vi "Control PID.vi"(5 "action":enum16{"CHECK", "INIT"}(ring), 6 "ITC temperature":dbl, 7 "time (sec)":dbl=3600.0, 8 "error in":errorcluster, 9 "Pid control":T1={" PID table "=[[400.0, 10.0, 3.0, 1.0], [300.0, 10.0, 3.0, 1.0], [60.0, 10.0, 3.0, 1.0], [40.0, 10.0, 3.0, 1.0], [20.0, 30.0, 0.5, 0.2], [10.0, 40.0, 0.5, 0.2], [1.0, 50.0, 0.2, 0.2], [0.0, 50.0, 0.2, 0.2]], "PID update interval (min)"=3600, "(mins) since PID update "=5.0, "P"=10.0, "I"=3.0, "D"=1.0, "PID is"=TRUE} {"D" format="%.2f"; "I" format="%.2f"; "P" format="%.2f"; "(mins) since PID update" format="%_3f"}) -> (0 "error out":errorcluster, 1 "Pid control Out":T1={" PID table "=[[400.0, 10.0, 3.0, 1.0], [300.0, 10.0, 3.0, 1.0], [60.0, 10.0, 3.0, 1.0], [40.0, 10.0, 3.0, 1.0], [20.0, 30.0, 0.5, 0.2], [10.0, 40.0, 0.5, 0.2], [1.0, 50.0, 0.2, 0.2], [0.0, 50.0, 0.2, 0.2]], "PID update interval (min)"=3600, "(mins) since PID update "=5.0, "P"=10.0, "I"=3.0, "D"=1.0, "PID is"=TRUE} {"D" format="%.2f"; "I" format="%.2f"; "P" format="%.2f"; "(mins) since PID update" format="%_3f"})   [LabVIEW 2012]
uses:
  Pid control.ctl
  itc 503 box - control.ctl
  Q -- check range -- i -- real.vi
  Q - not nan and gtr than zero - Real.vi
  Q - not nan -- real.vi
panel:
  # "Temp (K)                  P                          I                         D"
  # "Temp (K)                  P                          I                         D"
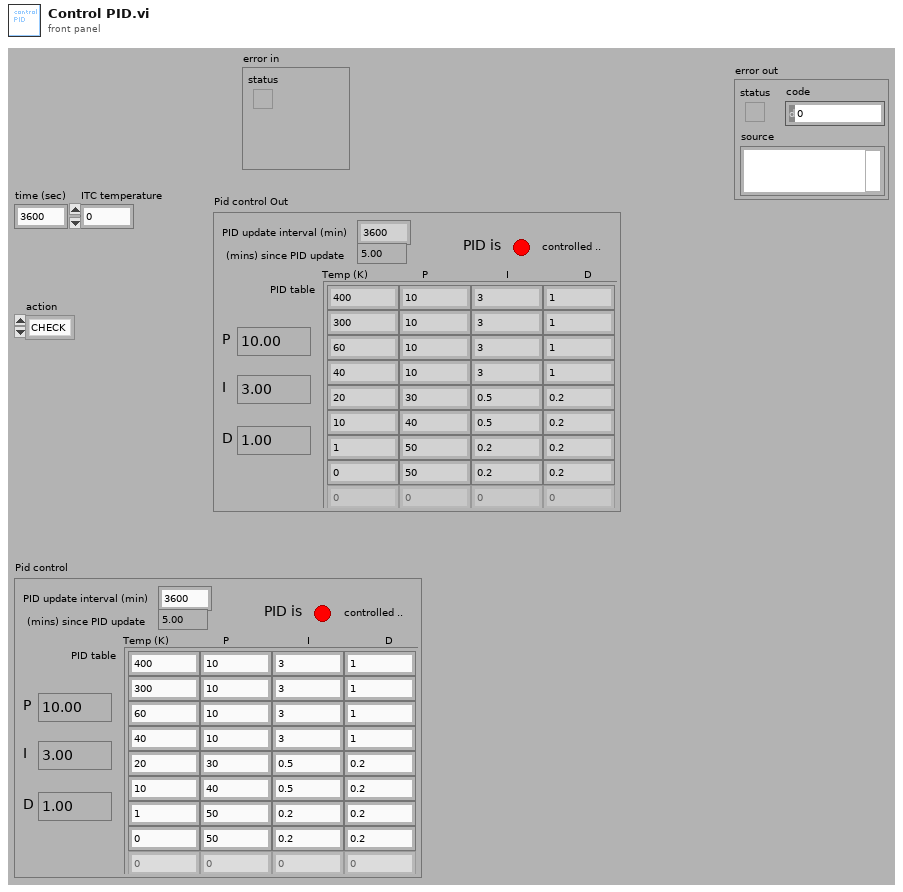
[diagram p1: front panel]
types:
  T1 = typedef "Pid control.ctl" = cluster{" PID table ":dbl[][], "PID update interval (min)":i32, "(mins) since PID update ":dbl, "P":dbl, "I":dbl, "D":dbl, "PID is":bool}
  T2 = typedef "itc 503 box - control.ctl" = enum16{"heater manual and zero", "heater auto", "upload D", "upload I", "upload P", "shut off", "init", "read sweep table", "disable", "enable", "read state", "set gas to", "stop sweep", "start sweep", "test", "set temperature to", "write sweep table"}
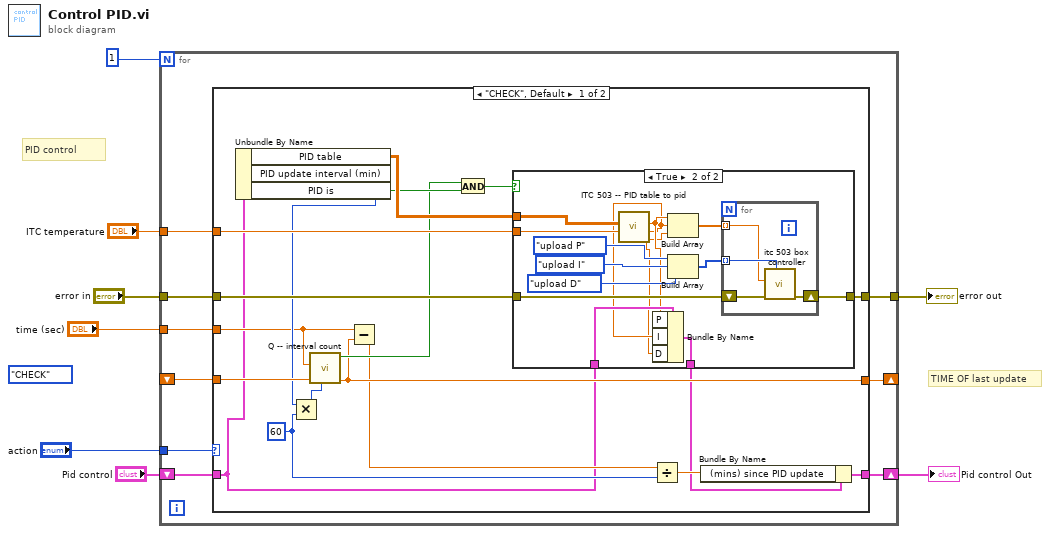
[diagram p0: block diagram]
diagram:
  (unwired) enum16{"CHECK", "INIT"}."CHECK" ("action")
  # "PID control"
  # "TIME OF last update"
  n1 = for {
    N: 1 -> [_]
    tunnel: "time (sec)" -> [w12]
    tunnel: "ITC temperature" -> [w17]
    tunnel: "error in" -> [w15]
    tunnel: [w14] -> w4
    shift-right: [w16] -> w6
    shift-left: "Pid control" -> [w13]
    tunnel: "action" -> [w11]
    shift-right: [w9] -> _
    shift-left: _ -> [w10]
    n2 = case shown="\"CHECK\", Default" w11 {
      tunnel: w17 -> [w34 _]
      tunnel: [w31 w56] -> w16
      tunnel: w15 -> [w29 w57]
      tunnel: [w28 w57] -> w14
      tunnel: w13 -> [w19 w56]
      tunnel: w12 -> [w22 w58]
      tunnel: w10 -> [w27 _]
      tunnel: [w21 w58] -> w9
      frame "CHECK", Default {
        w25 = 60
        n3 = Unbundle By Name(w19) -> ("PID table"=w33:dbl[][], "PID update interval (min)"=w26:i32, "PID is"=w32:bool)
        n4 = Multiply(x=w26, y=w25) -> (x*y=w24:i32)
        n5 = call "Q -- interval count.vi"("interval (sec)"=w24, "last time (sec)"=w27, "current time (sec)"=w22) -> ("last time out (sec)"=w21:dbl, "tic"=w23:bool)  [unwired: 5 in, 2 out]
        n6 = Subtract(x=w22, y=w21) -> (x-y=w20:dbl)
        n7 = And(x=w23, y=w32) -> (x .and. y?=w35:bool)
        n8 = case shown="True" w35 {
          tunnel: w33 -> [_ w51]
          tunnel: w34 -> [_ w50]
          tunnel: w29 -> [w37 w43]
          tunnel: [w37 w49] -> w28
          tunnel: w19 -> [w36 w42]
          tunnel: [w36 w41] -> w18
          frame False {
          }
          frame True {
            n9 = call "ITC 503 -- PID table to pid.vi"("temperature"=w50, "PID table"=w51) -> ("D"=w38:dbl, "I"=w39:dbl, "P"=w40:dbl)  [unwired: 7 in]
            n10 = Bundle By Name(cluster=w42, "P"=w40, "I"=w39, "D"=w38) -> (w41:T1)
            n11 = Build Array(w40, w39, w38) -> (w44:dbl[])
            n12 = Build Array(itc_503_box_-_control."upload P" ("itc box action"), itc_503_box_-_control."upload I" ("itc box action"), itc_503_box_-_control."upload D" ("itc box action")) -> (w45:T2[])
            n13 = for {
              tunnel: w45 -> [w54] mode=indexing
              tunnel: w44 -> [w53] mode=indexing
              shift-right: [w55] -> w49
              shift-left: w43 -> [w52]
              n14 = call "itc 503 box controller.vi"("itc box action"=w54, "error in"=w52, "input"=w53) -> ("error out"=w55:errorcluster)  [unwired: 6 in, 2 out]
            }
          }
        }
        n15 = Divide(x=w20, y=w25) -> (x/y=w30:dbl)
        n16 = Bundle By Name(cluster=w18, "(mins) since PID update"=w30) -> (w31:T1)
      }
      frame "INIT" {
      }
    }
  }
  "Pid control Out" <- w6
  "error out" <- w4
